vi "Sweep control recursive.vi"(6 "Experiment folder name":string="3- sweep Vsg_50mK_field", 8 "Comments":string="SA02704G.20140716\nbackgate=0V") -> ()   [LabVIEW 2013]
doc: "Instructions: \n1, you can put multiple scan names in one priority.\n2 OFF has to put in last priority"
uses:
  lockin/branches/PPMS-demomode-JL/Lockin-4461_MultiChannel - IV 3.0 globals.vi
panel:
  in  "Scan":T1(array[cluster])=[{"Scan control"=5, "Priority"=0, "Additional Action"=4, "Scan Parameters"={"DAQ Channel"=2, "Label"="scaledVsg1=", "Scaled low"=0.14, "Scaled high"=-0.06, "Start"=0.14, "End"=-0.06, "Step"=-0.06, "Scale?"=TRUE}, "OSC Configuration"={"Signal Type"=enum."Sine Wave", "DC"=0.0, "Amplitude"=0.2, "frequency"=20.0, "Phase"=0.0}}, {"Scan control"=1, "Priority"=0, "Additional Action"=4, "Scan Parameters"={"DAQ Channel"=0, "Label"="", "Scaled low"=0.0, "Scaled high"=0.0, "Start"=0.0, "End"=0.0, "Step"=0.0, "Scale?"=FALSE}, "OSC Configuration"={"Signal Type"=enum."Sine Wave", "DC"=0.0, "Amplitude"=0.2, "frequency"=20.0, "Phase"=0.0}}, {"Scan control"=1, "Priority"=0, "Additional Action"=4, "Scan Parameters"={"DAQ Channel"=0, "Label"="", "Scaled low"=0.0, "Scaled high"=0.0, "Start"=0.0, "End"=0.0, "Step"=0.0, "Scale?"=FALSE}, "OSC Configuration"={"Signal Type"=enum."Sine Wave", "DC"=0.0, "Amplitude"=0.2, "frequency"=20.0, "Phase"=0.0}}, {"Scan control"=1, "Priority"=0, "Additional Action"=4, "Scan Parameters"={"DAQ Channel"=0, "Label"="", "Scaled low"=0.0, "Scaled high"=0.0, "Start"=0.0, "End"=0.0, "Step"=0.0, "Scale?"=FALSE}, "OSC Configuration"={"Signal Type"=enum."Sine Wave", "DC"=0.0, "Amplitude"=0.2, "frequency"=20.0, "Phase"=0.0}}] {"OSC Configuration"."frequency" format="%0.2p"; "OSC Configuration"."Amplitude" format="%0.2p"; "OSC Configuration"."DC" format="%.2p"; "Scan Parameters"."Scaled low" format="%#_6p"; "Scan Parameters"."Scaled high" format="%#_6p"; "Scan Parameters"."Start" format="%#_6p"; "Scan Parameters"."End" format="%#_6p"; "Scan Parameters"."Step" format="%#_6p"; "Additional Action" items=["Clear DAQ Tasks", "Check Temperature", "Check Field Value", "Wait", "Do Nothing"]; "Priority" items=["Priority 0", "Priority 1", "Priority 2", "Priority 3", "Priority 4", "Priority 5"]; "Scan control" items=["OFF", "Vsg1", "Vsg2", "Vsgw", "Vbg", "Field", "Temp"]}
  in  "Number of IV curves":i32=1
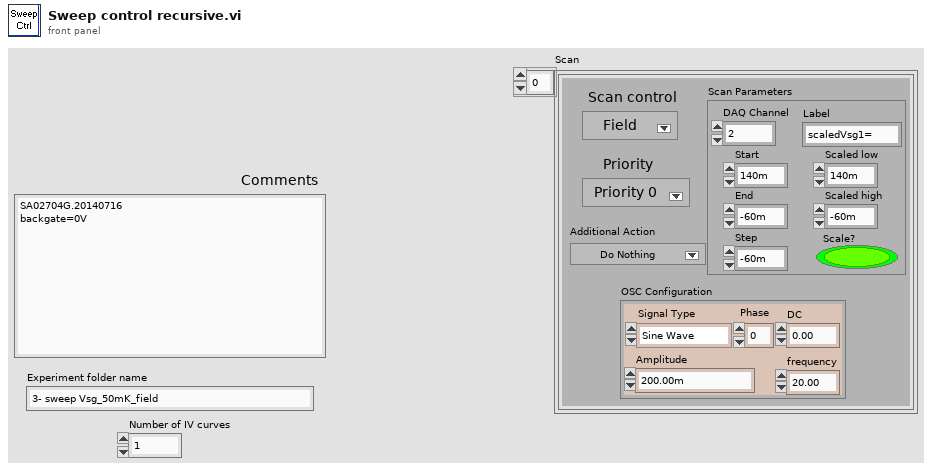
[diagram p1: front panel]
types:
  T1 = cluster{"Scan control":u16, "Priority":u16, "Additional Action":u16, "Scan Parameters":cluster{"DAQ Channel":i32, "Label":string, "Scaled low":dbl, "Scaled high":dbl, "Start":dbl, "End":dbl, "Step":dbl, "Scale?":bool}, "OSC Configuration":cluster{"Signal Type":enum16{"Sine Wave", "Triangle Wave", "Square Wave", "Sawtooth Wave"}, "DC":dbl, "Amplitude":dbl, "frequency":dbl, "Phase":dbl}}[]
  T2 = cluster{cluster{"DAQ Channel":i32, "Label":string, "Scaled low":dbl, "Scaled high":dbl, "Start":dbl, "End":dbl, "Step":dbl, "Scale?":bool}[]}[]
  T3 = cluster{cluster{"Priority":u16, "Scan name":u16}[]}[]
  T4 = cluster{cluster{"Priority":u16, "Scan name":u16}[]}
  T5 = cluster{cluster{"DAQ Channel":i32, "Label":string, "Scaled low":dbl, "Scaled high":dbl, "Start":dbl, "End":dbl, "Step":dbl, "Scale?":bool}[]}
  T6 = cluster{"DAQ Channel":i32, "Label":string, "Scaled low":dbl, "Scaled high":dbl, "Start":dbl, "End":dbl, "Step":dbl, "Scale?":bool}[]
  T7 = cluster{"Signal Type":enum16{"Sine Wave", "Triangle Wave", "Square Wave", "Sawtooth Wave"}, "DC":dbl, "Amplitude":dbl, "frequency":dbl, "Phase":dbl}[]
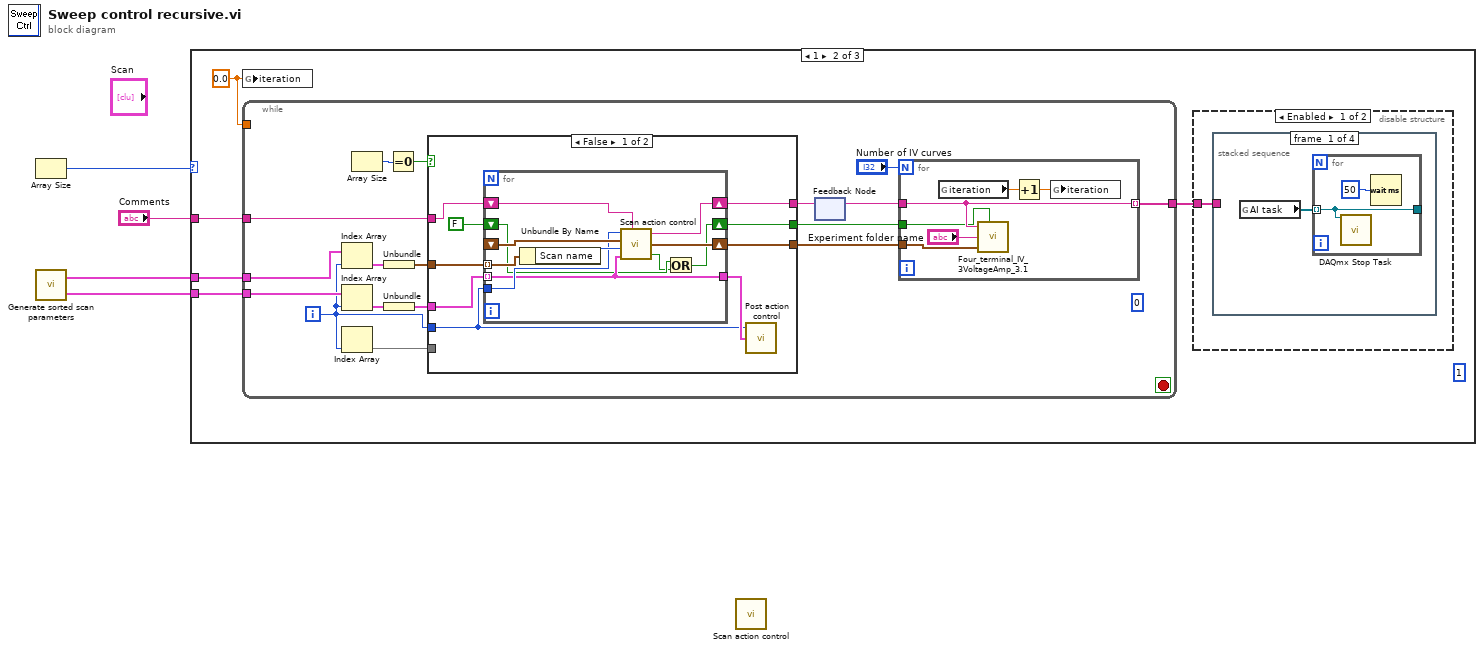
[diagram p0: block diagram]
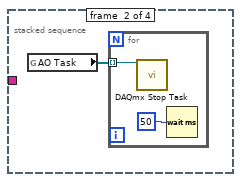
[diagram p3: hidden frame]
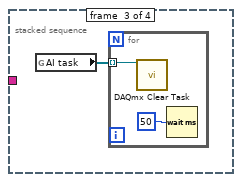
[diagram p4: hidden frame]
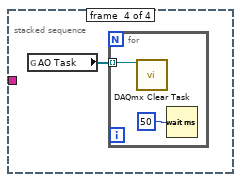
[diagram p5: hidden frame]
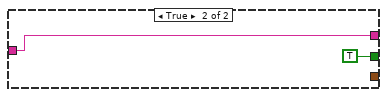
[diagram p7: hidden frame]
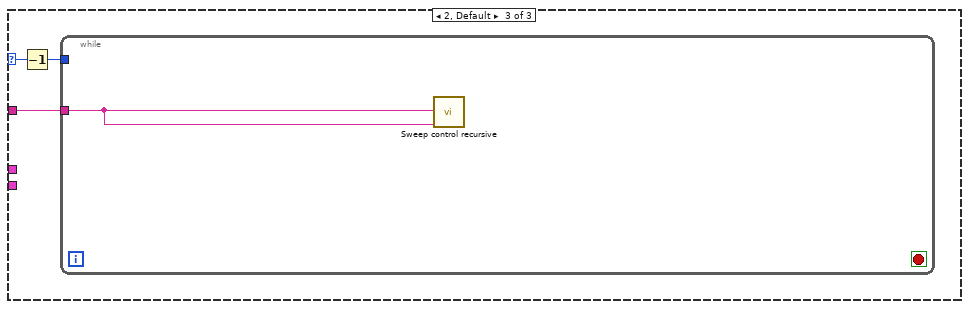
[diagram p8: hidden frame]
diagram:
  n1 = Array Size() -> (size(s)=w4:i32)  [unwired: 1 in]
  n2 = call "Generate sorted scan parameters.vi"() -> ("Sorted scan parameters"=w1:T2, "Sorted scan control"=w2:T3)  [unwired: 2 in]
  n3 = case shown="1" w4 {
    selector: w4 -> [_ _ w70]
    tunnel: "Comments" -> [_ w6 w68]
    tunnel: w2 -> [_ w7 _]
    tunnel: w1 -> [_ w5 _]
    frame 0 {
    }
    frame 1 {
      (unwired) 1
      w8 = 0.0 ("iteration")
      n4 = global write "Lockin-4461_MultiChannel - IV 3.0 globals.vi" "iteration"(w8) -> ()
      n5 = while {
        tunnel: w7 -> [w34]
        tunnel: w8 -> [_]
        tunnel: [w38] -> w9
        tunnel: w6 -> [w32]
        tunnel: w5 -> [w31]
        i -> [w30]
        stop <- _ stop-if-true
        (unwired) 0
        n6 = Index Array(array=w34, index=w30) -> (element=w35:T4)
        n7 = Index Array(array=w31, index=w30) -> (element=w29:T5)
        n8 = Index Array(index=w30) -> (element=w33)  [unwired: 1 in]
        n9 = Array Size() -> (size(s)=w37:i32)  [unwired: 1 in]
        n10 = Unbundle(w35) -> (w27:cluster{"Priority":u16, "Scan name":u16}[])
        n11 = Unbundle(w29) -> (w28:T6)
        n12 = Equal To 0?(x=w37) -> (x = 0?=w36:bool)
        n13 = case shown="False" w36 {
          tunnel: w28 -> [w48 _]
          tunnel: w32 -> [w47 w61]
          tunnel: [w46 _] -> w26
          tunnel: [w45 w61] -> w25
          tunnel: [w40 TRUE ("Stop?")] -> w23
          tunnel: w27 -> [w44 _]
          tunnel: w30 -> [w42 _]
          tunnel: w33 -> [_ _]
          frame False {
            n14 = for {
              tunnel: w44 -> [w59] mode=indexing
              tunnel: w48 -> [w52] mode=indexing
              tunnel: w42 -> [w53]
              shift-right: [w57] -> w46
              shift-left: _ -> [w56]
              shift-right: [w55] -> w45
              shift-left: w47 -> [w54]
              tunnel: [w52] -> w43
              shift-right: [w49] -> w40
              shift-left: FALSE -> [w51]
              n15 = Unbundle By Name(w59) -> ("Scan name"=w58:u16)
              n16 = call "Scan action control.vi"("Index"=w53, "OSC Configuration"=w56, "Scan control"=w58, "Scan Parameters"=w52, "Comments"=w54) -> ("Comments out"=w55:string, "OSC Configuration out"=w57:T7, "Stop?"=w50:bool)
              n17 = Or(x=w51, y=w50) -> (x .or. y?=w49:bool)
            }
            n18 = call "Post action control.vi"("Scan Parameters"=w43, "Index"=w42) -> ()  [unwired: 1 in, 1 out]
          }
          frame True {
          }
        }
        n19 = feedback-in #1(w25) -> ()
        n20 = feedback #1() -> (w24:string)  [unwired: 1 in]
        n21 = for {
          N: "Number of IV curves" -> [_]
          tunnel: w26 -> [w66]
          tunnel: [w63] -> w38 mode=indexing
          tunnel: w24 -> [w63]
          tunnel: w23 -> [w62]
          n22 = global read "Lockin-4461_MultiChannel - IV 3.0 globals.vi" "iteration"() -> (w65:dbl)
          n23 = call "Four_terminal_IV_3VoltageAmp_3.1.vi"("Comments"=w63, "Single IV curve?"=w62, "Experiment folder name"="Experiment folder name", "OSC Configuration"=w66) -> ()  [unwired: 5 out]
          n24 = Increment(x=w65) -> (x+1=w64:dbl)
          n25 = global write "Lockin-4461_MultiChannel - IV 3.0 globals.vi" "iteration"(w64) -> ()
        }
      }
      n26 = disable-structure shown="Enabled" {
        disable-tunnel: w9 -> [w10 _]
        frame Enabled {
          n27 = stacked-sequence {
            tunnel: w10 -> [_ _ _ _]
            frame #0 {
              n28 = global read "Lockin-4461_MultiChannel - IV 3.0 globals.vi" "AI task"() -> (w11:refnum<k21>[])
              n29 = for {
                tunnel: w11 -> [w12] mode=indexing
                tunnel: [w12] -> _
                n30 = call <vilib>:"DAQmx Stop Task.vi"("task/channels in"=w12) -> ()  [unwired: 13 in, 2 out]
                n31 = Wait (ms)(milliseconds to wait=u32 50) -> ()  [unwired: 1 out]
              }
            }
            frame #1 {
              n32 = global read "Lockin-4461_MultiChannel - IV 3.0 globals.vi" "AO Task"() -> (w14:refnum<k21>[])
              n33 = for {
                tunnel: w14 -> [w16] mode=indexing
                n34 = call <vilib>:"DAQmx Stop Task.vi"("task/channels in"=w16) -> ()  [unwired: 13 in, 2 out]
                n35 = Wait (ms)(milliseconds to wait=u32 50) -> ()  [unwired: 1 out]
              }
            }
            frame #2 {
              n36 = global read "Lockin-4461_MultiChannel - IV 3.0 globals.vi" "AI task"() -> (w17:refnum<k21>[])
              n37 = for {
                tunnel: w17 -> [w19] mode=indexing
                n38 = call <vilib>:"DAQmx Clear Task.vi"("task in"=w19) -> ()  [unwired: 14 in, 1 out]
                n39 = Wait (ms)(milliseconds to wait=u32 50) -> ()  [unwired: 1 out]
              }
            }
            frame #3 {
              n40 = global read "Lockin-4461_MultiChannel - IV 3.0 globals.vi" "AO Task"() -> (w20:refnum<k21>[])
              n41 = for {
                tunnel: w20 -> [w22] mode=indexing
                n42 = call <vilib>:"DAQmx Clear Task.vi"("task in"=w22) -> ()  [unwired: 14 in, 1 out]
                n43 = Wait (ms)(milliseconds to wait=u32 50) -> ()  [unwired: 1 out]
              }
            }
          }
        }
        frame Disabled {
        }
      }
    }
    frame 2, Default {
      n44 = Decrement(x=w70) -> (x-1=w69:i32)
      n45 = while {
        tunnel: w69 -> [_]
        tunnel: w68 -> [w71]
        stop <- _ stop-if-true
        n46 = call "Sweep control recursive.vi"("Experiment folder name"=w71, "Comments"=w71) -> ()  [unwired: 10 in]
      }
    }
  }
  n47 = call "Scan action control.vi"() -> ()  [unwired: 5 in, 3 out]
